vi "Position Main Pane Tab.vi"(8 "error in (no error)":errorcluster, 10 "This VI":refnum<vi>, 11 "Side Tab Ref":refnum<vi>) -> (0 "error out":errorcluster)   [LabVIEW 2014]
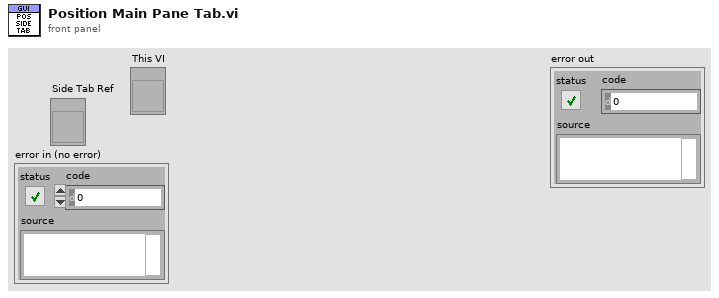
[diagram p1: front panel]
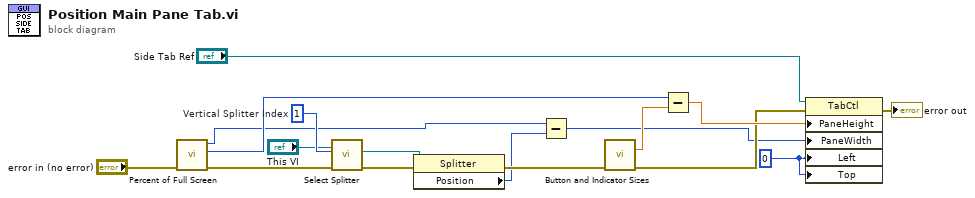
[diagram p0: block diagram]
diagram:
  w9 = 1  # Vertical Splitter Index
  w12 = 0 ("Position:Left")
  n1 = call "Percent of Full Screen.vi"("error in (no error)"="error in (no error)") -> ("error out"=w8:errorcluster, "Bottom"=w15:i16, "Right"=w4:i16)  [unwired: 8 in]
  n2 = call "Select Splitter.vi"("error in (no error)"=w8, "Pane Index"=w9, "This VI"="This VI") -> ("error out"=w6:errorcluster, "Splitter"=w7:refnum<vi>)  [unwired: 6 in, 1 out]
  n3 = property class="Splitter"(reference=w7, error in=w6) -> (error out=w5:errorcluster, "Position"=w3:i32)  [unwired: 1 out]
  n4 = Subtract(x=w4, y=w3) -> (x-y=w2:i32)
  n5 = call "Button and Indicator Sizes.vi"("error in (no error)"=w5) -> ("Button Height"=w14:dbl, "error out"=w11:errorcluster)  [unwired: 10 in, 3 out]
  n6 = Subtract(x=w15, y=w14) -> (x-y=w13:dbl)
  n7 = property class="TabCtl"(reference="Side Tab Ref", error in=w11, "PaneHeight"=w13, "PaneWidth"=w2, "Left"=w12, "Top"=w12) -> (error out=→"error out":errorcluster)  [unwired: 1 out]
